vi "DEPP Smart Enable.vi"(8 "Error In":errorcluster, 11 "Adept Config":T1) -> (0 "Error Out":errorcluster, 2 "Success?":bool, 3 "Adept Config":T1)   [LabVIEW 2011, in "LVH-Adept.lvlib"]
uses:
  LVH-Adept.lvlib
  Type Defs/Device Config.ctl
  Type Defs/Status.ctl
  DEPP/DEPP.lvlib
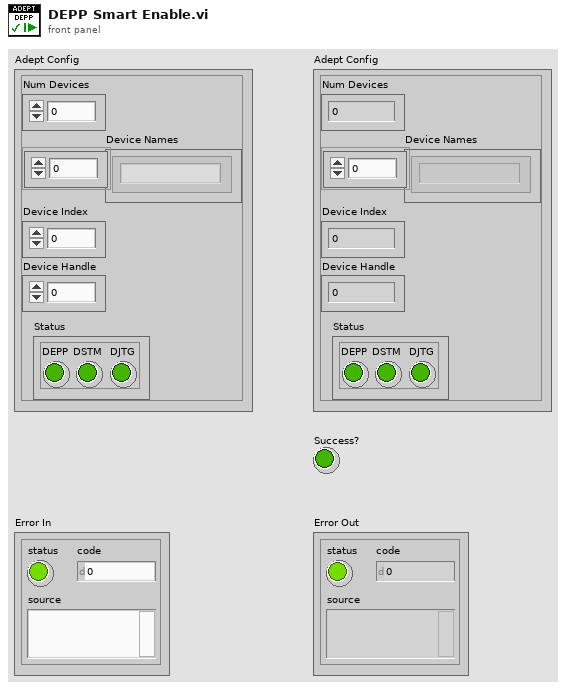
[diagram p1: front panel]
types:
  T1 = typedef "LVH-Adept.lvlib/Device Config.ctl" = cluster{"Num Devices":i32, "Device Names":string[], "Device Index":u16, "Device Handle":u32, "Status":T2}
  T2 = typedef "LVH-Adept.lvlib/Status.ctl" = cluster{"DEPP":bool, "DSTM":bool, "DJTG":bool}
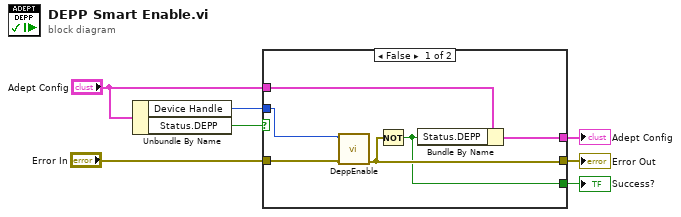
[diagram p0: block diagram]
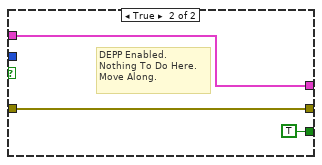
[diagram p2: hidden frame]
diagram:
  n1 = Unbundle By Name("Adept Config") -> ("Device Handle"=w6:u32, "Status.DEPP"=w7:bool)
  n2 = case shown="False" w7 {
    tunnel: w6 -> [w12 _]
    tunnel: "Error In" -> [w13 w16]
    tunnel: [w9 w16] -> w4
    tunnel: "Adept Config" -> [w11 w15]
    tunnel: [w10 w15] -> w2
    tunnel: [w8 TRUE] -> w1
    frame False {
      n3 = call "DeppEnable.vi"("Error In"=w13, "Device Handle"=w12) -> ("Error Out"=w9:errorcluster)  [unwired: 8 in, 1 out]
      n4 = Not(x=w9) -> (.not. x?=w8:bool)
      n5 = Bundle By Name(cluster=w11, "Status.DEPP"=w8) -> (w10:T1)
    }
    frame True {
      # "DEPP Enabled.\nNothing To Do Here.\nMove Along."
    }
  }
  "Error Out" <- w4
  "Adept Config" <- w2
  "Success?" <- w1
